vi "PID.vi"() -> ()   [LabVIEW 2021]
uses:
  <vilib>/Instr/_visa.llb/VISA Configure Serial Port (Instr).vi
panel:
  in  "STOP":bool
  in  "Start":bool
  out "Right":bool
  out "Left":bool
  in  "Setpint":dbl(slide)=8.0 min=8.0 max=60.0 step=1.0 scale=8.0..60.0
  out "Waveform":cluster{"Setpint":dbl, i32}(graph)
  in  "COM PORT":refnum<visa-resource-name>
  in  "stop":bool
  # "Set-Point"
  # "Distance"
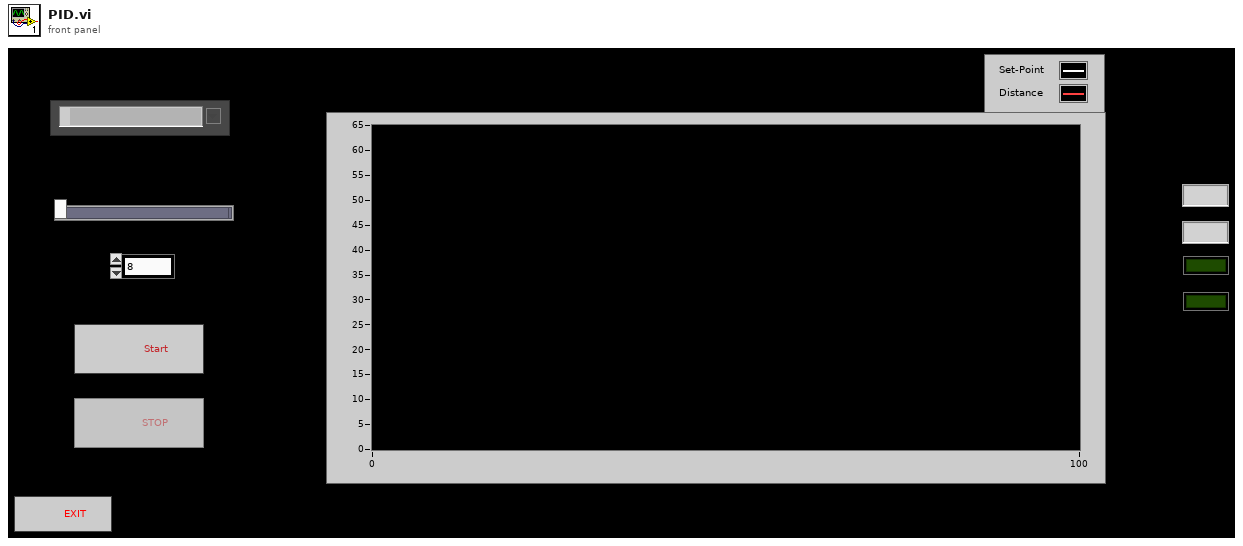
[diagram p1: front panel]
types:
  T1 = enum8{"Enabled", "Disabled", "Disabled and Grayed Out"}
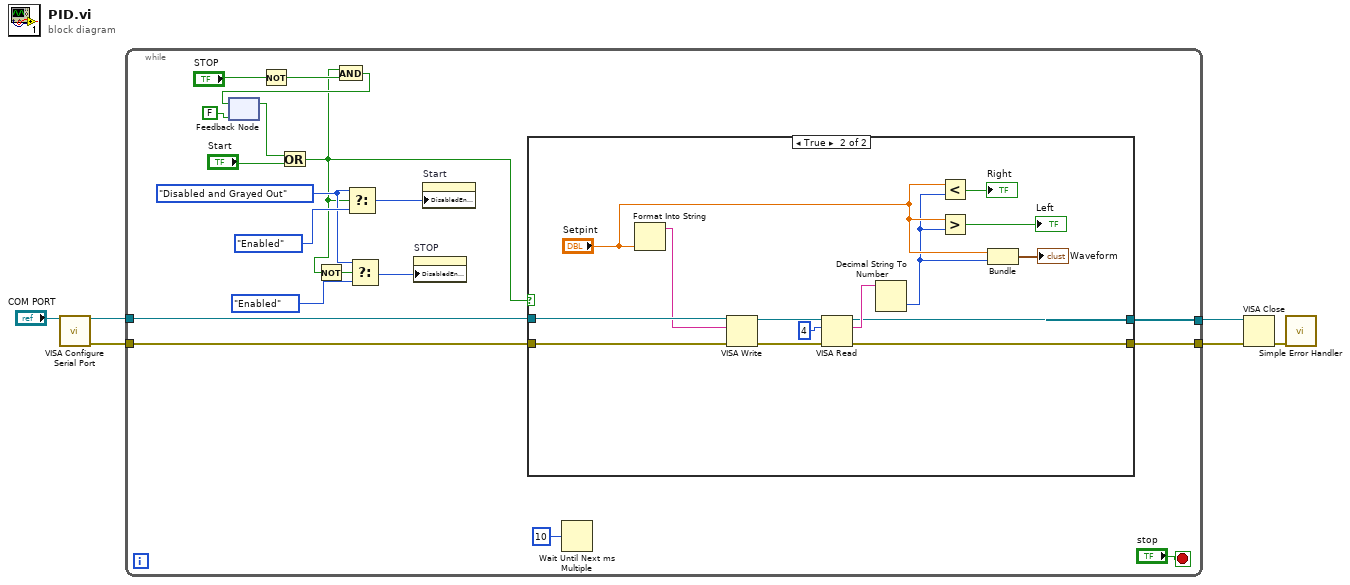
[diagram p0: block diagram]
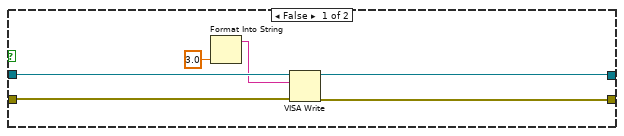
[diagram p2: hidden frame]
diagram:
  n1 = call-poly "VISA Configure Serial Port"("VISA resource name"="COM PORT") -> ("VISA resource name out"=w6:refnum<visa-resource-name>, "error out"=w5:errorcluster)  [unwired: 13 in]
  n2 = while {
    tunnel: w6 -> [w21]
    tunnel: w5 -> [w20]
    tunnel: [w23] -> w2
    tunnel: [w22] -> w1
    stop <- "stop" stop-if-true
    w11 = T1."Disabled and Grayed Out" ("t")
    n3 = feedback #1(FALSE) -> (w17:bool)
    n4 = Not(x="STOP") -> (.not. x?=w19:bool)
    n5 = Or(x=w17, y="Start") -> (x .or. y?=w7:bool)
    n6 = Not(x=w7) -> (.not. x?=w10:bool)
    n7 = And(x=w7, y=w19) -> (x .and. y?=w18:bool)
    n8 = feedback-in #1(w18) -> ()
    n9 = Select(t=w11, s=w7, f=T1."Enabled" ("Disabled")) -> (s? t:f=w12:T1)
    n10 = Select(t=w11, s=w10, f=T1."Enabled") -> (s? t:f=w8:T1)
    n11 = property on="STOP" class="Bool"("DisabledEnum"=w8) -> ()  [unwired: 2 in, 2 out]
    n12 = property on="Start" class="Bool"("DisabledEnum"=w12) -> ()  [unwired: 2 in, 2 out]
    n13 = case shown="True" w7 {
      tunnel: [w29 w43] -> w23
      tunnel: [w28 w42] -> w22
      tunnel: w21 -> [w31 w38]
      tunnel: w20 -> [w30 w37]
      frame False {
        n14 = Format Into String(3.0 ("input 1")) -> (resulting string=w26:string)  [unwired: 3 in, 1 out]
        n15 = VISA Write(VISA resource name=w31, write buffer=w26, error in (no error)=w30) -> (VISA resource name out=w29:refnum<visa-resource-name>, error out=w28:errorcluster)  [unwired: 1 out]
      }
      frame True {
        n16 = Format Into String("Setpint") -> (resulting string=w32:string)  [unwired: 3 in, 1 out]
        n17 = VISA Write(VISA resource name=w38, write buffer=w32, error in (no error)=w37) -> (VISA resource name out=w40:refnum<visa-resource-name>, error out=w39:errorcluster)  [unwired: 1 out]
        n18 = VISA Read(VISA resource name=w40, byte count=u32 4, error in (no error)=w39) -> (VISA resource name out=w43:refnum<visa-resource-name>, read buffer=w45:string, error out=w42:errorcluster)  [unwired: 1 out]
        n19 = Decimal String To Number(string=w45) -> (number=w34:i32)  [unwired: 2 in, 1 out]
        n20 = Less?(x="Setpint", y=w34) -> (x < y?=→"Right":bool)
        n21 = Greater?(x="Setpint", y=w34) -> (0:→"Left":bool)
        n22 = Bundle("Setpint"="Setpint", w34) -> (→"Waveform":cluster{"Setpint":dbl, i32})  [unwired: 1 in]
      }
    }
    n23 = Wait Until Next ms Multiple(millisecond multiple=u32 10 ("milliseconds to wait")) -> ()  [unwired: 1 out]
  }
  n24 = VISA Close(VISA resource name=w2, error in (no error)=w1) -> (error out=w4:errorcluster)
  n25 = call <vilib>:"Simple Error Handler.vi"("error in (no error)"=w4) -> ()  [unwired: 4 in, 5 out]
